vi "Day1_string.vi"() -> ()   [LabVIEW 2014]
panel:
  out "일치 + 문자열의 나머지":string
  out "일치 구문 앞 부분 문자열":string
  out "Required string":string
  out "String to number":dbl
  out "String subset":string
  out "String length":i32
  out "Cancatenated string":string
  in  "Input string":string
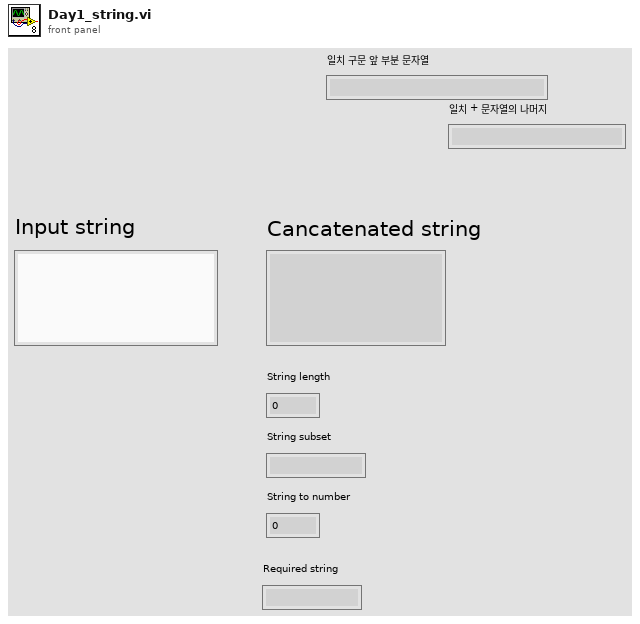
[diagram p1: front panel]
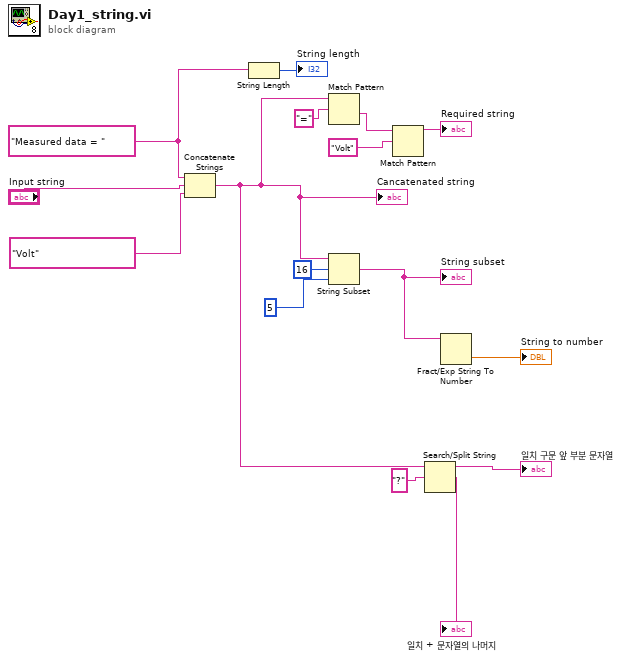
[diagram p0: block diagram]
diagram:
  w14 = "Measured data = "
  n1 = Concatenate Strings(w14, "Input string", "Volt") -> (w4:string)
  "Cancatenated string" <- w4
  n2 = String Length(string=w14) -> (length=→"String length":i32)
  n3 = Match Pattern(string=w4, regular expression="=") -> (after substring=w7:string)  [unwired: 1 in, 3 out]
  n4 = String Subset(string=w4, offset (0)=16 ("오프셋(0)"), length (rest)=5 ("길이(나머지)")) -> (substring=w10:string)
  "String subset" <- w10
  n5 = Match Pattern(string=w7, regular expression="Volt") -> (before substring=→"Required string":string)  [unwired: 1 in, 3 out]
  n6 = Search/Split String(string=w4, search string/char (-)="?" ("검색 문자열/문자 (-)")) -> (substring before match=→"일치 구문 앞 부분 문자열":string, match + rest of string=→"일치 + 문자열의 나머지":string)  [unwired: 1 in, 1 out]
  n7 = Fract/Exp String To Number(string=w10) -> (number=→"String to number":dbl)  [unwired: 3 in, 1 out]
